vi "Measure_C_F.vi"(5 "Junction Name":string, 6 "UiDefinition":T1, 7 ".NET Refnum":refnum<k24>, 8 "new file path (Not A Path if cancelled)":path, 10 "appended path":path, 11 ".NET Refnum in":refnum<k24>) -> (0 "error out":errorcluster, 3 "Cluster":cluster{dbl[], dbl[]})   [LabVIEW 2020]
uses:
  UIReferences.ctl
  C:/Users/User/Desktop/Automation/CurrentVersion/LabviewDXFViewer/bin/Release/LabviewDXFViewer.exe
  LabviewDXFViewer/bin/Release/LabviewDXFViewer.exe
  <vilib>/Analysis/6fits.llb/Curve Fitting Criteria.ctl
  <vilib>/Utility/file.llb/Write Delimited Spreadsheet (DBL).vi
  <vilib>/Utility/file.llb/Write Delimited Spreadsheet (string).vi
  <vilib>/Analysis/NI_AALPro.lvlib
panel:
  in  "CurrentPositionIndex":i32
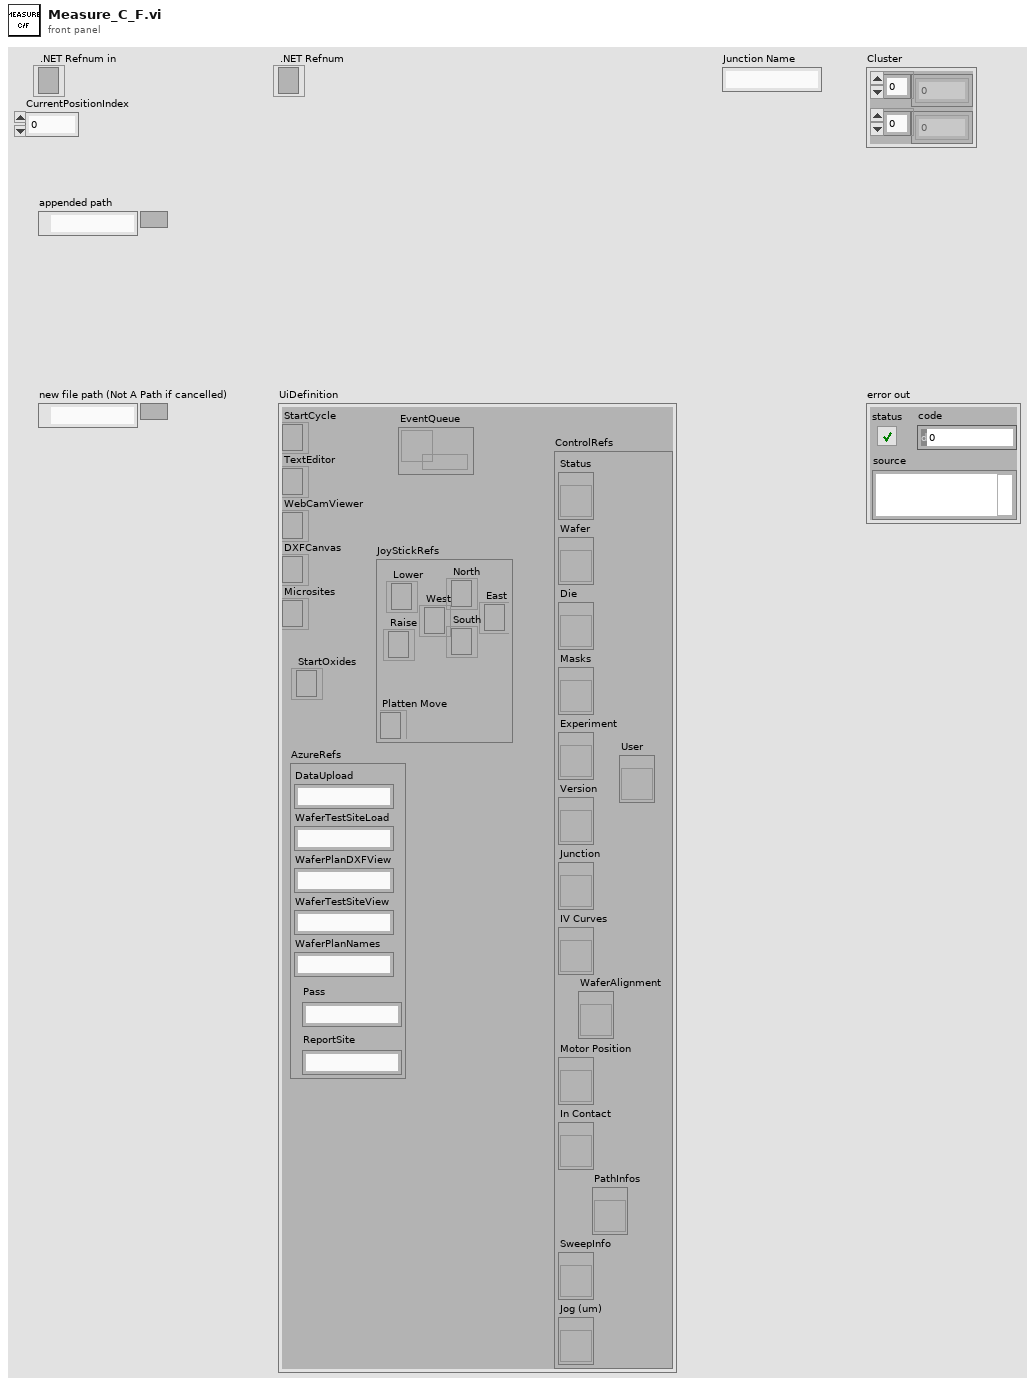
[diagram p1: front panel]
types:
  T1 = typedef "UIReferences.ctl" = cluster{"StartCycle":refnum<k24>, "TextEditor":refnum<k24>, "WebCamViewer":refnum<k24>, "DXFCanvas":refnum<k24>, "Microsites":refnum<k24>, "JoyStickRefs":cluster{"North":refnum<k24>, "Lower":refnum<k24>, "Raise":refnum<k24>, "Platten Move":refnum<k24>, "West":refnum<k24>, "East":refnum<k24>, "South":refnum<k24>}, "AzureRefs":cluster{"DataUpload":string, "WaferTestSiteLoad":string, "WaferPlanDXFView":string, "WaferTestSiteView":string, "WaferPlanNames":string, "Pass":string, "ReportSite":string}, "ControlRefs":cluster{"Status":refnum<vi>, "Wafer":refnum<vi>, "Die":refnum<vi>, "Masks":refnum<vi>, "Experiment":refnum<vi>, "Version":refnum<vi>, "Junction":refnum<vi>, "IV Curves":refnum<vi>, "Motor Position":refnum<vi>, "In Contact":refnum<vi>, "SweepInfo":refnum<vi>, "Jog (um)":refnum<vi>, "PathInfos":refnum<vi>, "User":refnum<vi>, "WaferAlignment":refnum<vi>}, "EventQueue":refnum<queue>, "StartOxides":refnum<k24>}
  T2 = typedef "NI_AALPro.lvlib/Curve Fitting Criteria.ctl" = u16
  T3 = typedef "CapacitanceInfos.ctl" = cluster{"Conductance":dbl, "CapacitanceIV":dbl, "Intercept":dbl, "CapacitanceSW":dbl, "Sum":dbl, "CapacitanceInfos":T4[], "CapacitancePhase":dbl, "dC/dV":dbl, "Function":string, "OtherInfo":dbl[][]}
  T4 = typedef "CapacitanceRecord.ctl" = cluster{"Freq":dbl, "Vpp":dbl, "PhaseS":dbl, "Irms":dbl, "PhaseC":dbl, "Theta":dbl, "VDrive":dbl, "Capacitance":dbl, "Other":dbl}
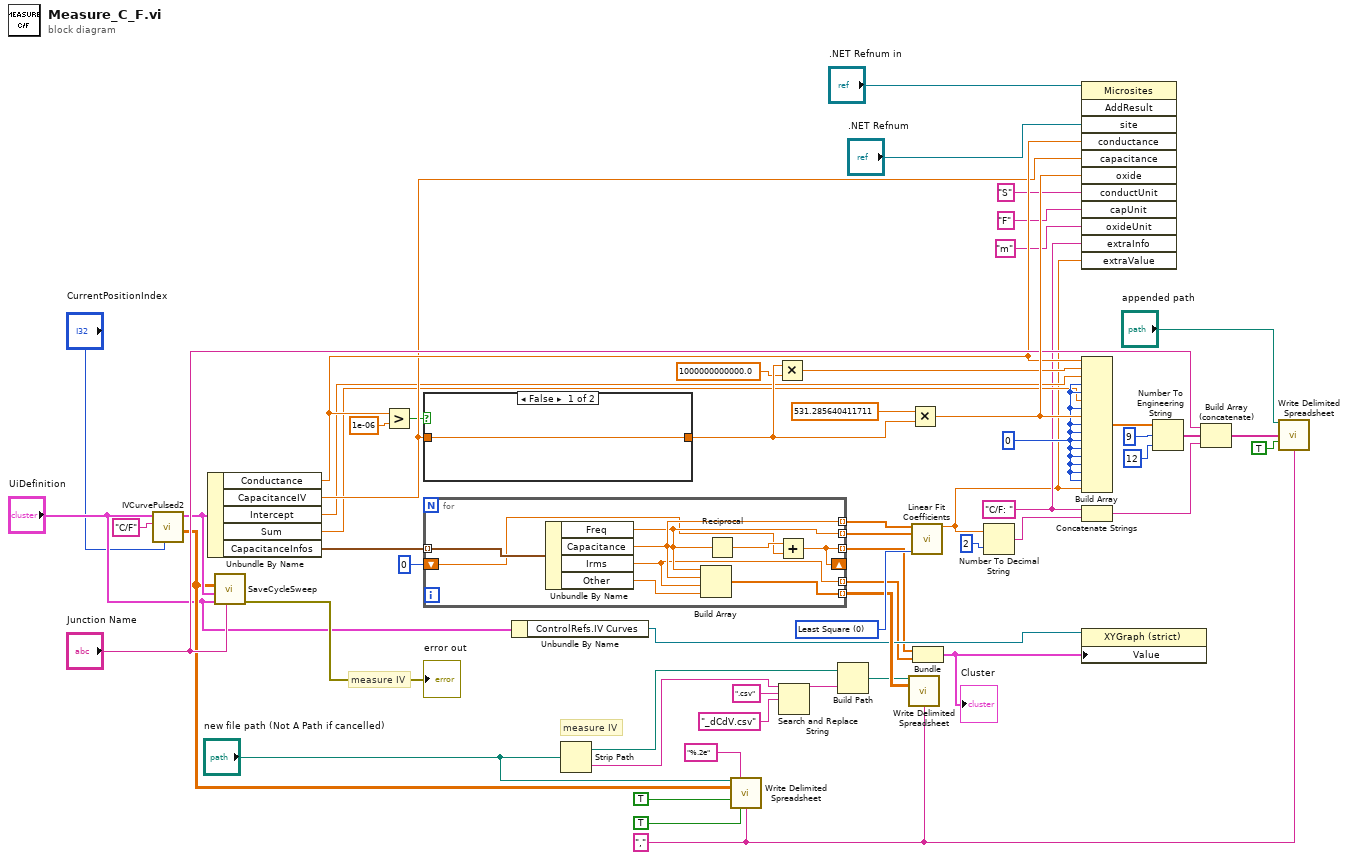
[diagram p0: block diagram]
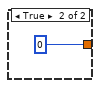
[diagram p2: hidden frame]
diagram:
  w3 = "C/F: "
  w13 = "," ("delimiter (\\t)")
  w51 = T2 0 items=["Least Square", "Least Absolute Residual", "Bisquare"] ("method")
  w52 = 0
  # "measure IV"
  # "measure IV"
  n1 = call "IVCurvePulsed2.vi"("CurrentPositionIndex"="CurrentPositionIndex", "Program"="C/F", "UiDefinition"="UiDefinition") -> ("appended array"=w30:dbl[][], "InfoCluster"=w43:T3)  [unwired: 7 in]
  n2 = Unbundle By Name(w43) -> ("Conductance"=w45:dbl, "CapacitanceIV"=w44:dbl, "Intercept"=w33:dbl, "Sum"=w34:dbl, "CapacitanceInfos"=w46:T4[])
  n3 = call "SaveCycleSweep.vi"("JunctionName"="Junction Name", "UiDefinition 2"="UiDefinition", "InfoCluster"=w43, "appended array"=w30) -> ("error out"=→"error out":errorcluster)  [unwired: 7 in]
  n4 = Greater?(x=w45, y=1e-06) -> (0:w37:bool)
  n5 = case shown="False" w37 {
    tunnel: [w58 0] -> w56
    tunnel: w44 -> [w58 _]
    frame False {
    }
    frame True {
    }
  }
  n6 = for {
    tunnel: w46 -> [w68] mode=indexing
    tunnel: [w65] -> w54 mode=indexing
    tunnel: [w67] -> w53 mode=indexing
    tunnel: [w66] -> w16 mode=indexing
    shift-right: [w62] -> _
    shift-left: 0 -> [w63]
    tunnel: [w62] -> w7 mode=indexing
    tunnel: [w61] -> w8 mode=indexing
    n7 = Unbundle By Name(w68) -> ("Freq"=w65:dbl, "Capacitance"=w67:dbl, "Irms"=w61:dbl, "Other"=w60:dbl)
    n8 = Build Array(w65, w67, w61, w60) -> (w66:dbl[])
    n9 = Reciprocal(x=w65) -> (1/x=w64:dbl)
    n10 = Add(x=w64, y=w63) -> (x+y=w62:dbl)
  }
  n11 = Unbundle By Name("UiDefinition") -> ("ControlRefs.IV Curves"=w11:refnum<vi>)
  n12 = Strip Path(path="new file path (Not A Path if cancelled)") -> (stripped path=w17:path, name=w21:string)
  n13 = call-poly <vilib>:"Write Delimited Spreadsheet.vi"("file path (dialog if empty)"="new file path (Not A Path if cancelled)", "format (%.3f)"="%.2e", "2D data"=w30, "append to file? (new file:F)"=TRUE, "transpose? (no:F)"=TRUE, "delimiter (\\t)"=w13) -> ()  [unwired: 8 in, 2 out]
  n14 = Multiply(x=w56, y=1000000000000.0) -> (x*y=w35:dbl)
  n15 = Search and Replace String(input string=w21, search string=".csv", replace string="_dCdV.csv" ("replace string (\"\")")) -> (result string=w18:string)  [unwired: 5 in, 3 out]
  n16 = Build Path(base path=w17, name or relative path=w18) -> (appended path=w14:path)
  n17 = call-poly <vilib>:"Write Delimited Spreadsheet.vi"("file path (dialog if empty)"=w14, "2D data"=w16, "delimiter (\\t)"=w13) -> ()  [unwired: 11 in, 2 out]
  n18 = Multiply(x=531.285640411711, y=w56) -> (x*y=w57:dbl)
  n19 = call <vilib>:"Linear Fit Coefficients.vi"("Y"=w53, "X"=w54, "method"=w51) -> ("slope"=w2:dbl)  [unwired: 10 in, 2 out]
  n20 = Bundle(w7, w8) -> (w10:cluster{dbl[], dbl[]})  [unwired: 1 in]
  "Cluster" <- w10
  n21 = Number To Decimal String(number=w2, width (-)=i16 2) -> (decimal integer string=w6:string)
  n22 = invoke class="Microsites" method="AddResult"(reference=".NET Refnum in", "site"=".NET Refnum", "conductance"=w45, "capacitance"=w44, "oxide"=w57, "conductUnit"="S", "capUnit"="F", "oxideUnit"="m" ("interceptUnit"), "extraInfo"=w3, "extraValue"=w2) -> ()  [unwired: 2 in, 12 out]
  n23 = Build Array(w45, w35, w33, w52, w52, w34, w52, w57, w52, w52, w52, w52, w52, w52, w52, w52, w2) -> (w32:dbl[])
  n24 = Concatenate Strings(w3, w6) -> (w4:string)
  n25 = property class="XYGraph (strict)"(reference=w11, "Value"=w10) -> ()  [unwired: 1 in, 2 out]
  n26 = Number To Engineering String(2:i16 12 ("precision (6)"), 3:i16 9 ("width (-)"), 4:w32) -> (0:w24:string[])  [unwired: 1 in]
  n27 = Build Array (concatenate)("Junction Name", w24, w4) -> (w26:string[])
  n28 = call-poly <vilib>:"Write Delimited Spreadsheet.vi"("file path (dialog if empty)"="appended path", "1D data"=w26, "append to file? (new file:F)"=TRUE, "delimiter (\\t)"=w13) -> ()  [unwired: 10 in, 2 out]
